vi "Day 1 solution.vi"() -> ()   [LabVIEW 2020]
uses:
  384769a4-19f5-4f83-a385-d88af59ea8e9.vi
  <vilib>/Comparison/Less/Less Functor/Less Functor.lvclass
panel:
  in  "Input":string="4514\n8009\n6703\n1811\n4881\n3905\n3933\n9436\n4332\n\n3059\n15715\n11597\n10625\n8486\n\n4556\n10613\n4087\n11287\n12020\n1412\n\n5320\n9757\n10646\n7373\n1197\n3486\n4359\n\n16319\n22687\n5272\n\n6167\n2478\n4950\n5513\n6113\n2739\n6805\n4488\n6555\n2752\n\n2198\n2528\n3432\n2218\n3283\n1400\n1932\n3438\n1834\n1050\n4766\n5218\n3033\n3410\n\n3362\n2773\n6782\n7416\n5388\n5419\n4628\n8877\n\n2852\n7531\n6028\n8068\n3942\n9388\n8053\n6334\n6099\n\n2086\n3097\n2914\n3087\n7500\n1718\n1482\n6198\n2057\n7098\n7464\n\n4522\n4306\n1906\n6692\n1273\n3851\n6475\n1186\n6012\n2456\n2414\n5740\n\n12352\n14613\n4339\n1259\n3363\n\n5505\n5913\n6539\n4164\n10864\n8085\n4962\n\n5427\n3232\n6945\n4536\n6549\n2299\n4450\n2130\n3757\n..."
  out "Sum of top 3 (Part 2)":i32
  out "max value (part 1)":i32
  # "Advent of code day 1"
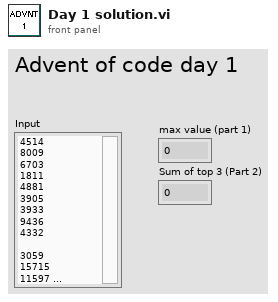
[diagram p1: front panel]
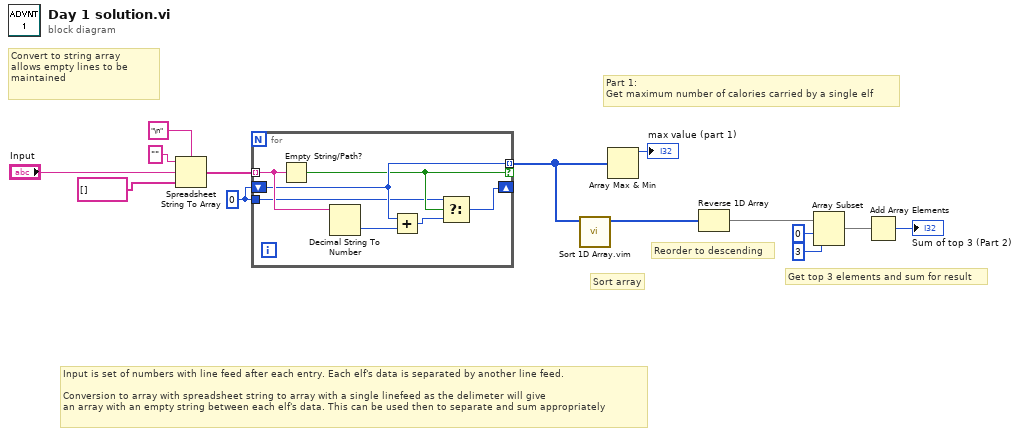
[diagram p0: block diagram]
diagram:
  w4 = 0
  # "Input is set of numbers with line feed after each entry. Each elf's data is separated by another line feed.\n\nConversion to array with spreadsheet string to array with a single linefeed as the delimeter will give \nan array with an empty string between each elf's data. This can be used then to separate and sum appropriately"
  # "Get top 3 elements and sum for result"
  # "Reorder to descending"
  # "Sort array"
  # "Part 1:\nGet maximum number of calories carried by a single elf"
  # "Convert to string array\nallows empty lines to be maintained"
  n1 = Spreadsheet String To Array(delimiter (Tab)="\n", format string="", spreadsheet string="Input", array type (2D Dbl)=string[] []) -> (array=w10:string[])
  n2 = for {
    tunnel: w10 -> [w21] mode=indexing
    shift-right: [w16] -> _
    shift-left: w4 -> [w19]
    tunnel: [w19] -> w3 mode=indexing if=w18
    tunnel: w4 -> [w15]
    n3 = Empty String/Path?(string/path=w21) -> (empty?=w18:bool)
    n4 = Decimal String To Number(string=w21) -> (number=w20:i32)  [unwired: 2 in, 1 out]
    n5 = Add(x=w19, y=w20) -> (x+y=w17:i32)
    n6 = Select(t=w15, s=w18, f=w17) -> (s? t:f=w16:i32)
  }
  n7 = call "Sort 1D Array.vim"("unsorted array"=w3) -> ("sorted array"=w2:i32[])  [unwired: 10 in]
  n8 = Array Max & Min(array=w3) -> (max value=→"max value (part 1)":i32)  [unwired: 3 out]
  n9 = Reverse 1D Array(array=w2) -> (reversed array=w1:i32[])
  n10 = Array Subset(array=w1, index=0, length=3) -> (w6:i32[])
  n11 = Add Array Elements(numeric array=w6) -> (sum=→"Sum of top 3 (Part 2)":i32)
